vi "RVHR_Export Results_ExaPromPDF.vi"(6 "Local Data":T1, 7 "appended path":path, 8 "error in (no error)":errorcluster, 11 "Feature Table":string[][](array[string])=[["T1_KGN-MMK_LeftRail_20221114__0000000000.jpeg", "L", "Corrugation", "0.011096", "0.002368", "0.011096", "0.002368"], ["T1_KGN-MMK_LeftRail_20221114__0000000000.jpeg", "L", "Unknown", "0.012672", "0.001415", "0.013120", "0.001978"], ["T1_KGN-MMK_LeftRail_20221114__0000000000.jpeg", "L", "Unknown", "0.009825", "0.001763", "0.010158", "0.002166"], ["T1_KGN-MMK_RightRail_20221114__0000000000.jpeg", "R", "Unknown", "0.011674", "0.001198", "0.011674", "0.001198"], ["T1_KGN-MMK_RightRail_20221114__0000000000.jpeg", "R", "Unknown", "0.009925", "0.000982", "0.010548", "0.001386"], ["T1_KGN-MMK_LeftRail_20221114__0000000000.jpeg", "L", "Unknown", "0.001140", "0.000809", "-0.000002", "-0.000002"], ["T1_KGN-MMK_LeftRail_20221114__0000000000.jpeg", "L", "Unknown", "0.015532", "0.000852", "0.015532", "0.000852"], ["T1_KGN-MMK_RightRail_20221114__0000000000.jpeg", "R", "Unknown", "0.012845", "0.000938", "0.013062", "0.001184"], ["T1_KGN-MMK_RightRail_20221114__0000000000.jpeg", "R", "Corrugation", "0.009232", "0.000896", "0.009723", "0.001315"], ["T1_KGN-MMK_RightRail_20221114__0001500000.jpeg", "R", "Corrugation", "0.305360", "0.001430", "0.305880", "0.001834"], ["T1_KGN-MMK_LeftRail_20221114__0000000000.jpeg", "L", "Corrugation", "0.010821", "0.001661", "0.011428", "0.002166"], ["T1_KGN-MMK_LeftRail_20221114__0000000000.jpeg", "L", "Unknown", "0.010158", "0.000634", "0.010619", "0.000982"], ["T1_KGN-MMK_RightRail_20221114__0002000000.jpeg", "R", "Unknown", "0.408032", "0.001069", "0.408495", "0.001632"], ["T1_KGN-MMK_LeftRail_20221114__0002500000.jpeg", "L", "Unknown", "0.515705", "0.001372", "0.516241", "0.001863"], ["T1_KGN-MMK_RightRail_20221114__0002200000.jpeg", "R", "Unknown", "0.453206", "0.001140", "0.452628", "0.000867"]]) -> (0 "error out":errorcluster)   [LabVIEW 2024]
uses:
  Controls/RVHR - Local Data.ctl
  Controls/Test Cluster.ctl
  Controls/Excluded Information.ctl
  Controls/Language.ctl
  Controls/Device_Type.ctl
  <vilib>/Utility/miscctls.llb/LVRectTypeDef.ctl
  <vilib>/Utility/miscctls.llb/LVBoundsTypeDef.ctl
  <vilib>/Exaprom PDF/Controls/Initialization Controls/Captions.ctl
  <vilib>/Exaprom PDF/Controls/Initialization Controls/Image or Table Caption.ctl
  <vilib>/Exaprom PDF/Controls/Font Controls/Font complete cluster.ctl
  <vilib>/Exaprom PDF/Controls/Font Controls/Font size.ctl
  <vilib>/Exaprom PDF/Controls/Font Controls/Font color.ctl
  <vilib>/Exaprom PDF/Controls/Font Controls/Type and encoding.ctl
  <vilib>/Exaprom PDF/Controls/Text Controls/Unicode/Type and run direction.ctl
  <vilib>/Exaprom PDF/Controls/Initialization Controls/At the opening.ctl
  <vilib>/Exaprom PDF/Controls/Initialization Controls/Defaut Paragraphe and Line Spacing.ctl
  <vilib>/Exaprom PDF/Controls/Text Controls/Texte alignement.ctl
  <vilib>/Exaprom PDF/Controls/Text Controls/Line spacing.ctl
  <vilib>/Exaprom PDF/Controls/Page Controls/Page setup.ctl
  <vilib>/Exaprom PDF/Controls/Page Controls/Page size.ctl
  <vilib>/Exaprom PDF/Controls/Page Controls/Page Orientation.ctl
  <vilib>/Exaprom PDF/Controls/Page Controls/Page Layout Custom.ctl
  <vilib>/Exaprom PDF/Controls/Page Controls/Page margins.ctl
  <vilib>/Exaprom PDF/Controls/Initialization Controls/PDF Details.ctl
  <vilib>/Exaprom PDF/Controls/Initialization Controls/File Permission Parameters.ctl
  <vilib>/Exaprom PDF/Controls/Header, Footer and Watermark Controls/Header or Footer.ctl
  <vilib>/Exaprom PDF/Controls/Header, Footer and Watermark Controls/Header or Footer Line cluster.ctl
  <vilib>/Exaprom PDF/Controls/Header, Footer and Watermark Controls/Header Footer Line.ctl
  <vilib>/Exaprom PDF/Controls/Initialization Controls/Unit.ctl
  <vilib>/Exaprom PDF/Controls/Header, Footer and Watermark Controls/Header or Footer  Image cluster.ctl
  <vilib>/Exaprom PDF/Controls/Table Controls/Cell Alignment 20px.ctl
  <vilib>/Exaprom PDF/Controls/Table Controls/Table properties.ctl
  <vilib>/Exaprom PDF/Controls/Table Controls/Table position.ctl
  <vilib>/Exaprom PDF/Controls/Header, Footer and Watermark Controls/Header or Footer  Text cluster.ctl
  <vilib>/Exaprom PDF/Controls/Font Controls/Font complete cluster horizontal.ctl
  <vilib>/Exaprom PDF/Controls/Header, Footer and Watermark Controls/Header or Footer  Page # cluster.ctl
  <vilib>/Exaprom PDF/Controls/Header, Footer and Watermark Controls/Page number.ctl
  <vilib>/Exaprom PDF/Controls/Table Controls/Table Appearance and Font Row [ ].ctl
  <vilib>/Exaprom PDF/Controls/Table Controls/One Row Appearance.ctl
  <vilib>/Exaprom PDF/Controls/Table Controls/Row from to.ctl
  <vilib>/Exaprom PDF/Controls/Table Controls/Cell, Alignment, LS and Font - hide Vmerge.ctl
  <vilib>/Exaprom PDF/Controls/Table Controls/Cell Type, Alignment and LS.ctl
  <vilib>/Exaprom PDF/Controls/Table Controls/Text vertical arrangement.ctl
  <vilib>/Exaprom PDF/Controls/Table Controls/Cell Appearance.ctl
  <vilib>/Exaprom PDF/Controls/Table Controls/Cell Border 20 px.ctl
  <vilib>/Exaprom PDF/Controls/Table Controls/Merge Horizontal.ctl
  <vilib>/Exaprom PDF/Controls/Table Controls/Merge Vertical.ctl
  <vilib>/Exaprom PDF/VIs/Low level/Header, Footer and Watermark Low level/Append Text HF.vi
  <vilib>/Exaprom PDF/VIs/Low level/Header, Footer and Watermark Low level/AppendLine seperator.vi
  <vilib>/Exaprom PDF/VIs/Low level/Header, Footer and Watermark Low level/Append Image HF.vi
  <vilib>/Exaprom PDF/VIs/Low level/Header, Footer and Watermark Low level/Append Page number HF.vi
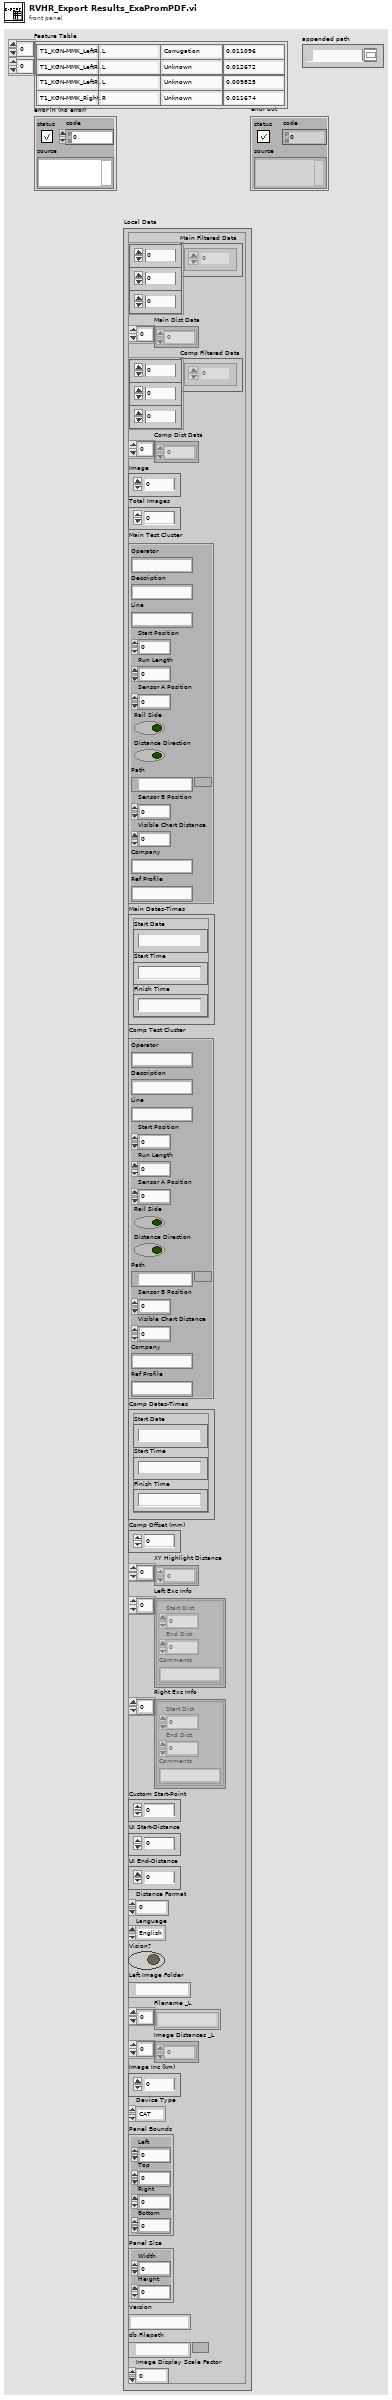
[diagram p1: front panel]
types:
  T1 = typedef "RVHR - Local Data.ctl" = cluster{"Main Filtered Data":dbl[][][], "Main Dist Data":dbl[], "Comp Filtered Data":dbl[][][], "Comp Dist Data":dbl[], "Image":u16, "Total Images":u16, "Main Test Cluster":T2, "Main Dates-Times":cluster{"Start Date":string, "Start Time":string, "Finish Time":string}, "Comp Test Cluster":T2, "Comp Dates-Times":cluster{"Start Date":string, "Start Time":string, "Finish Time":string}, "Comp Offset (mm)":i64, "XY Highlight Distance":dbl[], "Left Exc Info":T3[], "Right Exc Info":T3[], "Custom Start-Point":dbl, "UI Start-Distance":dbl, "UI End-Distance":dbl, "Distance Format":u8, "Language":T4, "Vision?":bool, "Left Image Folder":path, "Filename _L":string[], "Image Distances _L":dbl[], "Image Inc (km)":dbl, "Device Type":T5, "Panel Bounds":T6, "Panel Size":T7, "Version":string, "db Filepath":path, "Image Display Scale Factor":dbl}
  T2 = typedef "Test Cluster.ctl" = cluster{"Operator":string, "Description":string, "Line":string, "Start Position":dbl, "Run Length":dbl, "Sensor A Position":dbl, "Rail Side":bool, "Distance Direction":bool, "Path":path, "Sensor B Position":dbl, "Visible Chart Distance":dbl, "Company":string, "Ref Profile":string}
  T3 = typedef "Excluded Information.ctl" = cluster{"Start Dist":dbl, "End Dist":dbl, "Comments":string}
  T4 = typedef "Language.ctl" = enum16{"English", "Chinese", "German"}
  T5 = typedef "Device_Type.ctl" = enum16{"CAT", "Bi-CAT", "YRCA", "RCA", "RV-HR", "TV-HR"}
  T6 = typedef "LVRectTypeDef.ctl" = cluster{"Left":i16, "Top":i16, "Right":i16, "Bottom":i16}
  T7 = typedef "LVBoundsTypeDef.ctl" = cluster{"Width":u32, "Height":u32}
  T8 = typedef "Table Appearance and Font Row [ ].ctl" = T9[]
  T9 = typedef "One Row Appearance.ctl" = cluster{"Row":T10, "Cell [ ]":T11[]}
  T10 = typedef "Row from to.ctl" = cluster{"From #":i16, "to #":i16}
  T11 = typedef "Cell, Alignment, LS and Font - hide Vmerge.ctl" = cluster{"Text":T12, "Cell Appearance":T16, "HMerge":T18, "VMerge":T19, "Font":T20}
  T12 = typedef "Cell Type, Alignment and LS.ctl" = cluster{"Cell Alignment":T13, "Text rotation":T14, "Line spacing":T15}
  T13 = typedef "Cell Alignment 20px.ctl" = u16
  T14 = typedef "Text vertical arrangement.ctl" = enum16{"None", "Clockwise", "Counterclockwise"}
  T15 = typedef "Line spacing.ctl" = enum16{"Select", "1.0", "1.5", "2.0"}
  T16 = typedef "Cell Appearance.ctl" = cluster{"Border":T17, "Thickness":sgl, "Color":u32, "BG":u32}
  T17 = typedef "Cell Border 20 px.ctl" = u16
  T18 = typedef "Merge Horizontal.ctl" = cluster{"From":i8, "to":i8}
  T19 = typedef "Merge Vertical.ctl" = cluster{"From":i8, "to":i8}
  T20 = typedef "Font complete cluster.ctl" = cluster{"Name":string, "Size":T21, "Color":T22, "Style":cluster{"Bold":bool, "Italic":bool, "Underline":bool, "Strikeout":bool}, "Type":T23}
  T21 = typedef "Font size.ctl" = sgl
  T22 = typedef "Font color.ctl" = u32
  T23 = typedef "Type and encoding.ctl" = cluster{"Type&direction":T24, "Embedded":bool, "Encoding":string}
  T24 = typedef "Type and run direction.ctl" = enum16{"Select", "ASCII", "UTF-16", "UTF-16 (default)", "UTF-16 (LTR)", "UTF-16 (RTL)"}
  T25 = typedef "Table properties.ctl" = cluster{"Table position":T26, "SpacingBefore (points)":sgl, "SpacingAfter (points)":sgl}
  T26 = typedef "Table position.ctl" = i32
  T27 = typedef "Header or Footer  Text cluster.ctl" = cluster{"Start at page":i32, "Cell Alignment":T13, "Line spacing":T15, "Text":string, "Font complete":T28, "Link":string}
  T28 = typedef "Font complete cluster horizontal.ctl" = cluster{"Name":string, "Size":T21, "Color":T22, "Style":cluster{"Bold":bool, "Italic":bool, "Underline":bool, "Strikeout":bool}, "Type":T23}
  T29 = typedef "Header or Footer  Page # cluster.ctl" = cluster{"Start at page":i32, "Start with #":i32, "Cell Alignment":T13, "Page #":T30, "Font":T28}
  T30 = typedef "Page number.ctl" = cluster{"Text 1":string, "Text 2":string, "Text 3":string}
  T31 = typedef "Header or Footer.ctl" = enum16{"Header", "Footer"}
  T32 = typedef "Header or Footer  Image cluster.ctl" = cluster{"Start at page":i32, "Cell Alignment":T13, "Path":path, "Image (%)":sgl, "Link":string}
  T33 = typedef "Unit.ctl" = enum16{"inch", "mm"}
  T34 = typedef "Header or Footer Line cluster.ctl" = cluster{"H/F Line":T35, "Thickness (point)":sgl, " Colour":u32}
  T35 = typedef "Header Footer Line.ctl" = enum16{"No line", "Horizontal line"}
  T36 = typedef "File Permission Parameters.ctl" = cluster{"User Password":string, "Owner Password":string, "Printing":enum16{"Allow Printing", "Allow Degraded Printing", "Don't Allow Printing"}, "Allow Modify Contents":bool, "Allow Copy":bool, "Allow Modify Annotations":bool, "Allow Fill In ":bool, "Allow Screen Readers":bool, "Allow Assembly":bool}
  T37 = typedef "PDF Details.ctl" = cluster{"Title":string, "Author":string, "Subject":string, "Keywords":string, "Creator":string}
  T38 = typedef "Page setup.ctl" = cluster{"Page Size":T39, "Orientation":T40, "Custom Size":T41, "Margins":T42}
  T39 = typedef "Page size.ctl" = i32
  T40 = typedef "Page Orientation.ctl" = enum16{"Portrait", "Landscape"}
  T41 = typedef "Page Layout Custom.ctl" = cluster{"Width":sgl, "Height":sgl}
  T42 = typedef "Page margins.ctl" = cluster{"Left":sgl, "Right":sgl, "Top":sgl, "Bottom":sgl}
  T43 = typedef "Defaut Paragraphe and Line Spacing.ctl" = cluster{" Aligment":T44, "Line spacing":T15}
  T44 = typedef "Texte alignement.ctl" = enum16{"Select", "CENTER", "JUSTIFY", "LEFT", "RIGHT"}
  T45 = typedef "At the opening.ctl" = cluster{"Page":u16, "Show Bookmarks":bool}
  T46 = typedef "Captions.ctl" = cluster{"Figure":T47, "Table":T47, "Font":T20}
  T47 = typedef "Image or Table Caption.ctl" = cluster{"Caption":string, "Separator":string, "Position":enum16{"Above", "Below"}}
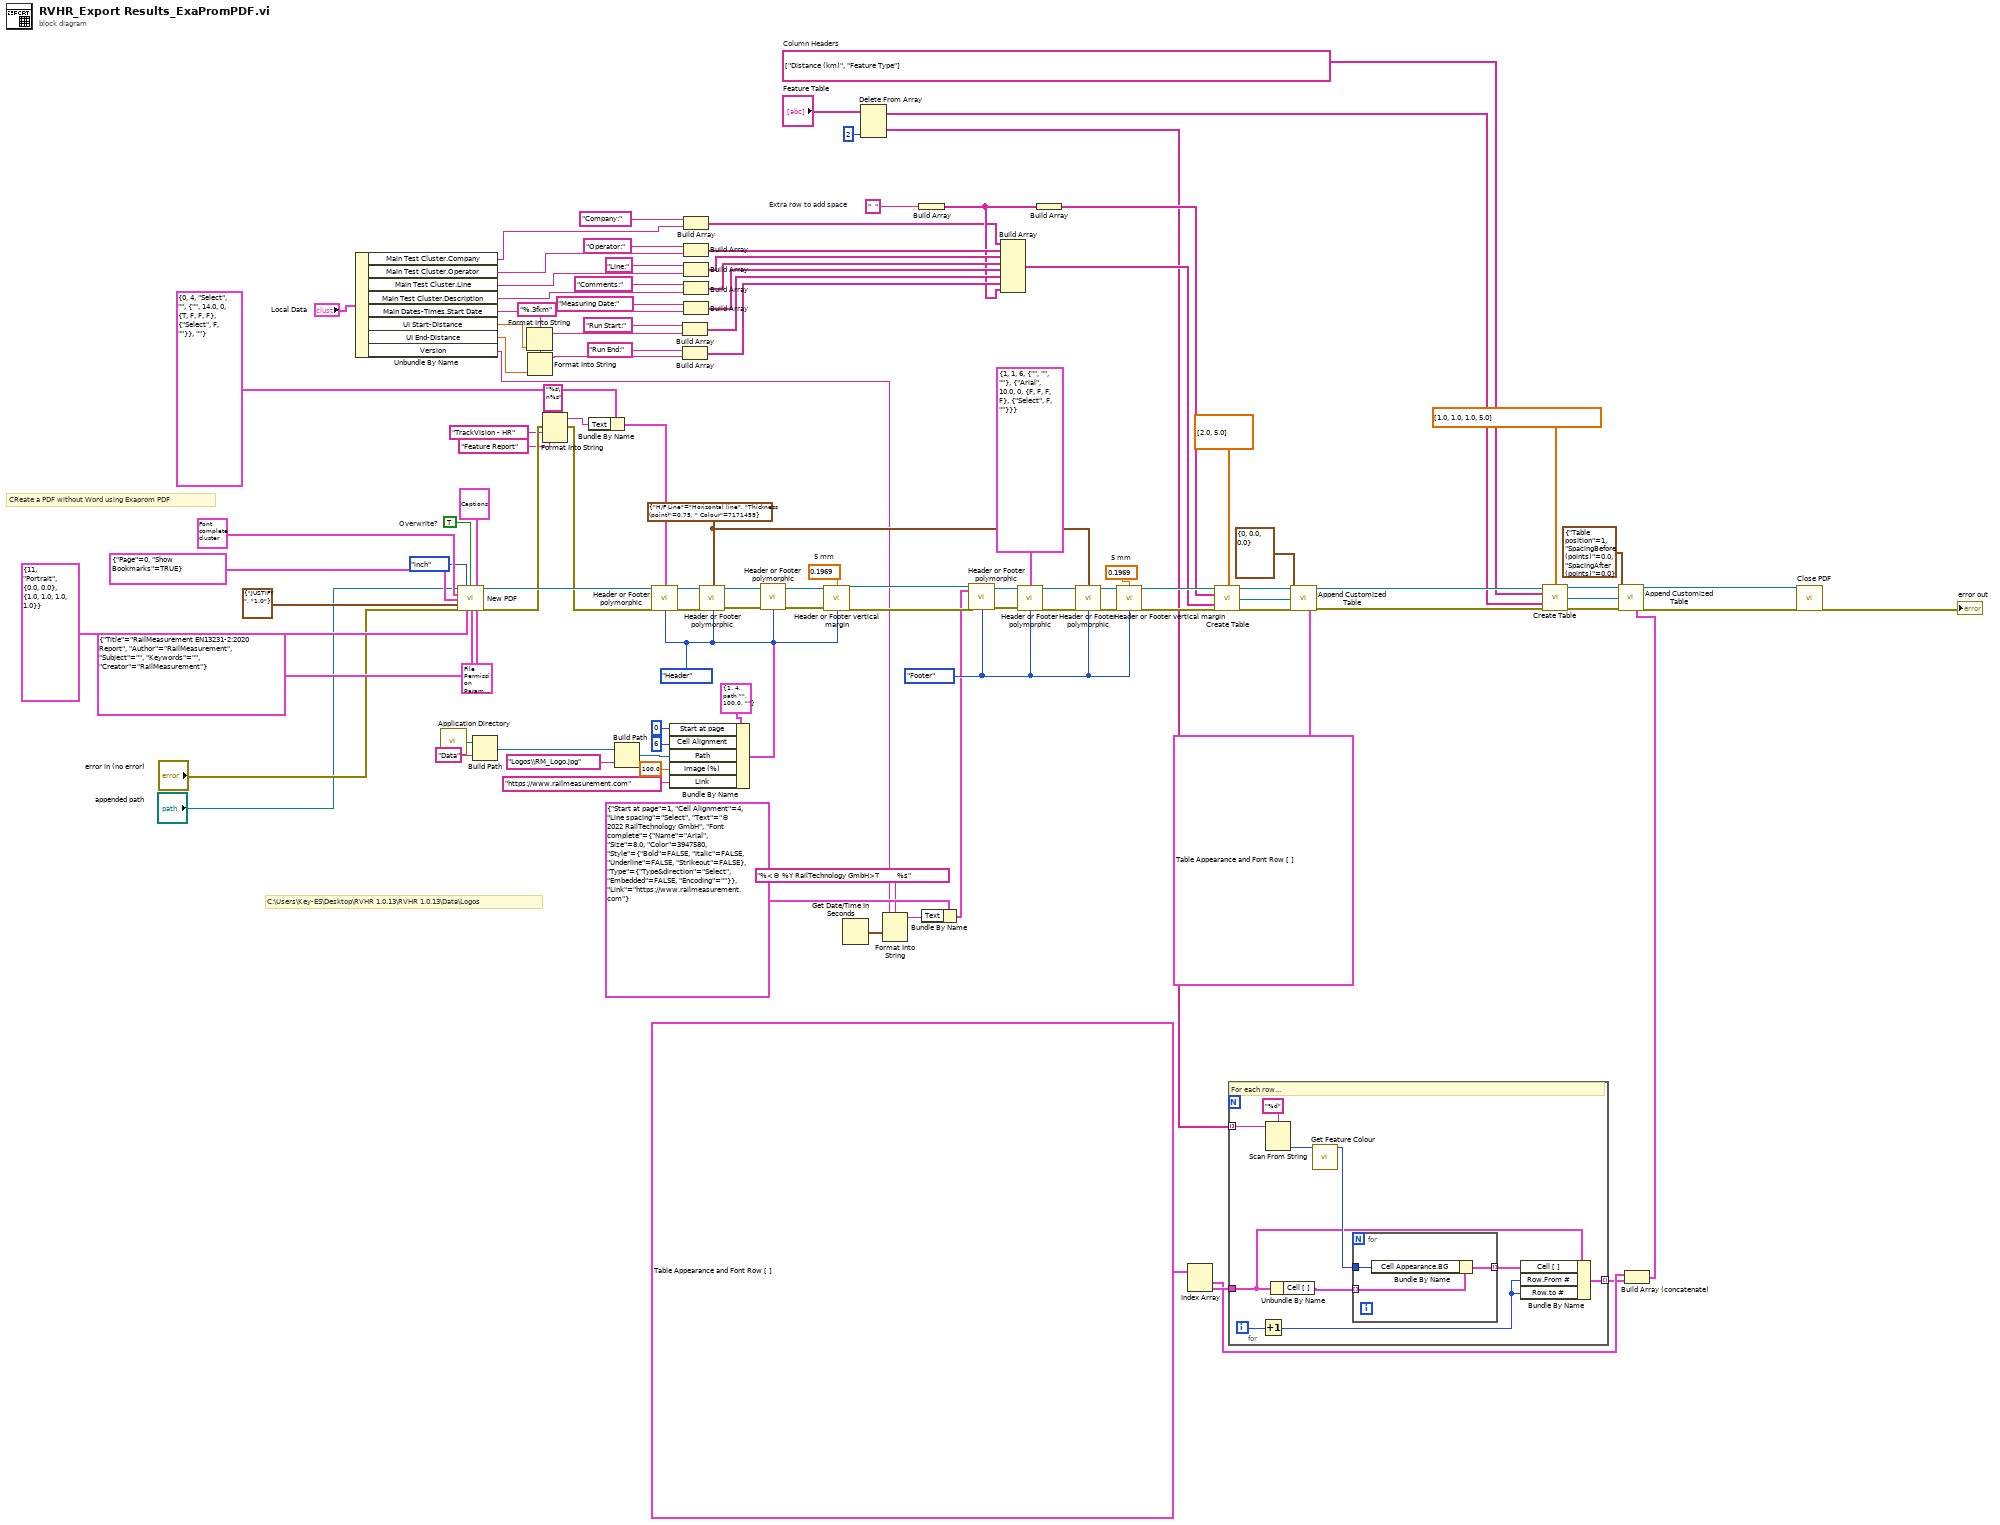
[diagram p0: block diagram]
diagram:
  w15 = "%.3fkm" ("format string")
  w26 = string[][] [["Distance (km)", "Feature Type"]]  # Column Headers
  w66 = "  "  # Extra row to add space
  w81 = 0.1969  # 5 mm
  w58 = Header_or_Footer."Footer" ("Position")
  w73 = T34 {"H/F Line"=enum."Horizontal line", "Thickness (point)"=0.75, " Colour"=7171459} ("Header Line")
  w105 = 0.1969  # 5 mm
  w96 = Header_or_Footer."Header" ("Position")
  w114 = TRUE  # Overwrite?
  # "C:\\Users\\Key-ES\\Desktop\\RVHR 1.0.13\\RVHR 1.0.13\\Data\\Logos"
  # "CReate a PDF without Word using Exaprom PDF"
  n1 = Unbundle By Name("Local Data") -> ("Main Test Cluster.Company"=w2:string, "Main Test Cluster.Operator"=w23:string, "Main Test Cluster.Line"=w22:string, "Main Test Cluster.Description"=w21:string, "Main Dates-Times.Start Date"=w20:string, "UI Start-Distance"=w19:dbl, "UI End-Distance"=w18:dbl, "Version"=w14:string)
  n2 = call <vilib>:"Application Directory.vi"() -> ("Application Directory"=w4:path)
  n3 = call <vilib>:"New PDF.vi"("PDF Path"="appended path", "Unit (default = mm)"=Unit."inch", "Overwrite?"=w114, "Captions"=T46 {"Figure"={"Caption"="Figure", "Separator"="  ", "Position"=enum."Below"}, "Table"={"Caption"="Table", "Separator"="  ", "Position"=enum."Above"}, "Font"={"Name"="", "Size"=-1.0, "Color"=0, "Style"={"Bold"=FALSE, "Italic"=FALSE, "Underline"=FALSE, "Strikeout"=FALSE}, "Type"={"Type&direction"=enum."Select", "Embedded"=FALSE, "Encoding"=""}}}, "Default Font"=T20 {"Name"="Arial", "Size"=12.0, "Color"=0, "Style"={"Bold"=FALSE, "Italic"=FALSE, "Underline"=FALSE, "Strikeout"=FALSE}, "Type"={"Type&direction"=enum."ASCII", "Embedded"=FALSE, "Encoding"=""}}, "At the opening"=T45 {"Page"=0, "Show Bookmarks"=TRUE}, "Default Paragraph"=T43 {" Aligment"=enum."JUSTIFY", "Line spacing"=enum."1.0"}, "error in (no error)"="error in (no error)", "Page Setup"=T38 {"Page Size"=11, "Orientation"=enum."Portrait", "Custom Size"={"Width"=0.0, "Height"=0.0}, "Margins"={"Left"=1.0, "Right"=1.0, "Top"=1.0, "Bottom"=1.0}}, "PDF Details"=T37 {"Title"="RailMeasurement EN13231-2:2020 Report", "Author"="RailMeasurement", "Subject"="", "Keywords"="", "Creator"="RailMeasurement"}, "Permissions"=T36 {"User Password"="", "Owner Password"="", "Printing"=enum."Allow Printing", "Allow Modify Contents"=TRUE, "Allow Copy"=TRUE, "Allow Modify Annotations"=TRUE, "Allow Fill In "=TRUE, "Allow Screen Readers"=TRUE, "Allow Assembly"=TRUE}) -> ("PDF Report"=w102:refnum<class "PDF Report Class.lvclass">, "error out"=w68:errorcluster)  [unwired: 3 out]
  n4 = Build Path(base path=w4, name or relative path="Data") -> (appended path=w90:path)
  n5 = Format Into String(format string=w15, w19) -> (resulting string=w16:string)  [unwired: 2 in, 1 out]
  n6 = Format Into String(format string=w15, w18) -> (resulting string=w17:string)  [unwired: 2 in, 1 out]
  n7 = Format Into String(format string="%s\n%s", error in=w68, "TrackVision - HR" ("input 1"), "Feature Report" ("input 2")) -> (resulting string=w71:string, error out=w67:errorcluster)  [unwired: 1 in]
  n8 = Bundle By Name(cluster=T27 {"Start at page"=0, "Cell Alignment"=4, "Line spacing"=enum."Select", "Text"="", "Font complete"={"Name"="", "Size"=14.0, "Color"=0, "Style"={"Bold"=TRUE, "Italic"=FALSE, "Underline"=FALSE, "Strikeout"=FALSE}, "Type"={"Type&direction"=enum."Select", "Embedded"=FALSE, "Encoding"=""}}, "Link"=""} ("Header Text"), "Text"=w71) -> (w69:T27)
  n9 = Build Path(base path=w90, name or relative path="Logos\\RM_Logo.jpg") -> (appended path=w53:path)
  n10 = call-poly <vilib>:"Header or Footer polymorphic.vi"("PDF Report IN"=w102, "Header or footer"=w69, "error in (no error)"=w67, "Position"=w96) -> ("PDF Report OUT"=w104:refnum<class "PDF Report Class.lvclass">, "error out"=w103:errorcluster)  [unwired: 10 out]
  n11 = Bundle By Name(cluster=T32 {"Start at page"=1, "Cell Alignment"=4, "Path"=path "", "Image (%)"=100.0, "Link"=""} ("Header or footer"), "Start at page"=0, "Cell Alignment"=T13 6, "Path"=w53, "Image (%)"=sgl 100.0, "Link"="https://www.railmeasurement.com") -> (w94:T32)
  n12 = Build Array("Run Start:" ("element"), w16) -> (w42:string[])
  n13 = Build Array("Run End:" ("element"), w17) -> (w41:string[])
  n14 = Build Array("Company:" ("element"), w2) -> (w1:string[])
  n15 = Build Array("Operator:" ("element"), w23) -> (w48:string[])
  n16 = Build Array("Line:" ("element"), w22) -> (w46:string[])
  n17 = Build Array("Comments:" ("element"), w21) -> (w47:string[])
  n18 = Build Array("Measuring Date:" ("element"), w20) -> (w43:string[])
  n19 = call-poly <vilib>:"Header or Footer polymorphic.vi"("PDF Report IN"=w104, "H/F Line"=w73, "error in (no error)"=w103, "Position"=w96) -> ("PDF Report OUT"=w100:refnum<class "PDF Report Class.lvclass">, "error out"=w99:errorcluster)  [unwired: 1 in, 9 out]
  n20 = call-poly <vilib>:"Header or Footer polymorphic.vi"("PDF Report IN"=w100, "Header or footer"=w94, "error in (no error)"=w99, "Position"=w96) -> ("PDF Report OUT"=w97:refnum<class "PDF Report Class.lvclass">, "error out"=w98:errorcluster)  [unwired: 1 in, 9 out]
  n21 = call <vilib>:"Header or Footer vertical margin.vi"("PDF Report IN"=w97, "Vertical margin"=w105, "error in (no error)"=w98, "Position"=w96) -> ("PDF Report OUT"=w62:refnum<class "PDF Report Class.lvclass">, "error out"=w61:errorcluster)  [unwired: 10 out]
  n22 = Get Date/Time In Seconds() -> (seconds since 1Jan1904=w54:timestamp)
  n23 = Delete From Array(array="Feature Table", index (col)=2 ("disabled index (col)")) -> (deleted portion=w5:string[], array with subset deleted=w6:string[][])  [unwired: 2 in]
  n24 = Format Into String(format string="%<© %Y RailTechnology GmbH>T         %s", w54, w14) -> (resulting string=w55:string)  [unwired: 2 in, 1 out]
  n25 = Build Array(w66) -> (w25:string[])
  n26 = Bundle By Name(cluster=T27 {"Start at page"=1, "Cell Alignment"=4, "Line spacing"=enum."Select", "Text"="© 2022 RailTechnology GmbH", "Font complete"={"Name"="Arial", "Size"=8.0, "Color"=3947580, "Style"={"Bold"=FALSE, "Italic"=FALSE, "Underline"=FALSE, "Strikeout"=FALSE}, "Type"={"Type&direction"=enum."Select", "Embedded"=FALSE, "Encoding"=""}}, "Link"="https://www.railmeasurement.com"} ("Footer Text"), "Text"=w55) -> (w57:T27)
  n27 = call-poly <vilib>:"Header or Footer polymorphic.vi"("PDF Report IN"=w62, "Header or footer"=w57, "error in (no error)"=w61, "Position"=w58) -> ("PDF Report OUT"=w59:refnum<class "PDF Report Class.lvclass">, "error out"=w60:errorcluster)  [unwired: 10 out]
  n28 = Build Array(w1, w48, w46, w47, w43, w42, w41, w25) -> (w40:string[][])
  n29 = call-poly <vilib>:"Header or Footer polymorphic.vi"("PDF Report IN"=w59, "Header or footer"=T29 {"Start at page"=1, "Start with #"=1, "Cell Alignment"=6, "Page #"={"Text 1"="", "Text 2"="", "Text 3"=""}, "Font"={"Name"="Arial", "Size"=10.0, "Color"=0, "Style"={"Bold"=FALSE, "Italic"=FALSE, "Underline"=FALSE, "Strikeout"=FALSE}, "Type"={"Type&direction"=enum."Select", "Embedded"=FALSE, "Encoding"=""}}} ("Footer Page #"), "error in (no error)"=w60, "Position"=w58) -> ("PDF Report OUT"=w77:refnum<class "PDF Report Class.lvclass">, "error out"=w76:errorcluster)  [unwired: 10 out]
  n30 = Build Array(w25) -> (w65:string[][])
  n31 = call-poly <vilib>:"Header or Footer polymorphic.vi"("PDF Report IN"=w77, "H/F Line"=w73, "error in (no error)"=w76, "Position"=w58) -> ("PDF Report OUT"=w74:refnum<class "PDF Report Class.lvclass">, "error out"=w75:errorcluster)  [unwired: 1 in, 9 out]
  n32 = call <vilib>:"Header or Footer vertical margin.vi"("PDF Report IN"=w74, "Vertical margin"=w81, "error in (no error)"=w75, "Position"=w58) -> ("PDF Report OUT"=w78:refnum<class "PDF Report Class.lvclass">, "error out"=w79:errorcluster)  [unwired: 10 out]
  n33 = Index Array(array=T8 [{"Row"={"From #"=0, "to #"=0}, "Cell [ ]"=[{"Text"={"Cell Alignment"=5, "Text rotation"=enum."None", "Line spacing"=enum."Select"}, "Cell Appearance"={"Border"=5, "Thickness"=0.5, "Color"=0, "BG"=16777225}, "HMerge"={"From"=-1, "to"=-1}, "VMerge"={"From"=-1, "to"=-1}, "Font"={"Name"="", "Size"=10.0, "Color"=0, "Style"={"Bold"=TRUE, "Italic"=FALSE, "Underline"=FALSE, "Strikeout"=FALSE}, "Type"={"Type&direction"=enum."Select", "Embedded"=FALSE, "Encoding"=""}}}, {"Text"={"Cell Alignment"=5, "Text rotation"=enum."None", "Line spacing"=enum."Select"}, "Cell Appearance"={"Border"=5, "Thickness"=0.5, "Color"=0, "BG"=16777225}, "HMerge"={"From"=-1, "to"=-1}, "VMerge"={"From"=-1, "to"=-1}, "Font"={"Name"="", "Size"=10.0, "Color"=0, "Style"={"Bold"=TRUE, "Italic"=FALSE, "Underline"=FALSE, "Strikeout"=FALSE}, "Type"={"Type&direction"=enum."Select", "Embedded"=FALSE, "Encoding"=""}}}]}, {"Row"={"From #"=1, "to #"=-1}, "Cell [ ]"=[{"Text"={"Cell Alignment"=5, "Text rotation"=enum."None", "Line spacing"=enum."Select"}, "Cell Appearance"={"Border"=5, "Thickness"=0.5, "Color"=0, "BG"=16777225}, "HMerge"={"From"=-1, "to"=-1}, "VMerge"={"From"=-1, "to"=-1}, "Font"={"Name"="", "Size"=10.0, "Color"=0, "Style"={"Bold"=FALSE, "Italic"=FALSE, "Underline"=FALSE, "Strikeout"=FALSE}, "Type"={"Type&direction"=enum."Select", "Embedded"=FALSE, "Encoding"=""}}}, {"Text"={"Cell Alignment"=5, "Text rotation"=enum."None", "Line spacing"=enum."Select"}, "Cell Appearance"={"Border"=5, "Thickness"=0.5, "Color"=0, "BG"=16777225}, "HMerge"={"From"=-1, "to"=-1}, "VMerge"={"From"=-1, "to"=-1}, "Font"={"Name"="", "Size"=10.0, "Color"=0, "Style"={"Bold"=FALSE, "Italic"=FALSE, "Underline"=FALSE, "Strikeout"=FALSE}, "Type"={"Type&direction"=enum."Select", "Embedded"=FALSE, "Encoding"=""}}}]}] ("Row  [ ]")) -> (element #1=w11:T9, element #2=w12:T9)  [unwired: 2 in]
  n34 = call <vilib>:"Create Table.vi"("PDF Report IN"=w78, "Table columnWidth [ ]"=sgl[] [2.0, 5.0], "Column Headers 2D [ ]"=w65, "Text Data 2D [ ]"=w40, "error in (no error)"=w79) -> ("PDF Report duplicate"=w84:refnum<class "PDF Report Class.lvclass">, "PDF Table"=w85:refnum<class "Pdfp Table Class.lvclass">, "error out"=w86:errorcluster)  [unwired: 8 in]
  n35 = for {
    tunnel: w12 -> [w116]
    tunnel: [w115] -> w10 mode=indexing
    tunnel: w5 -> [w123] mode=indexing
    i -> [w118]
    # "For each row..."
    n36 = Increment(x=w118) -> (x+1=w117:i32)
    n37 = Scan From String(format string="%d", input string=w123) -> (output 1=w122:u16)  [unwired: 3 in, 3 out]
    n38 = Unbundle By Name(w116) -> ("Cell [ ]"=w121:T11[])
    n39 = call "Get Feature Colour.vi"("Feature Type"=w122) -> ("color"=w120:u32)  [unwired: 10 in]
    n40 = for {
      tunnel: w121 -> [w127] mode=indexing
      tunnel: w120 -> [w126]
      tunnel: [w125] -> w119 mode=indexing
      n41 = Bundle By Name(cluster=w127, "Cell Appearance.BG"=w126) -> (w125:T11)
    }
    n42 = Bundle By Name(cluster=w116, "Cell [ ]"=w119, "Row.From #"=w117, "Row.to #"=w117) -> (w115:T9)
  }
  n43 = call <vilib>:"Append Customized Table.vi"("PDF Report IN"=w84, "Table properties"=T25 {"Table position"=0, "SpacingBefore (points)"=0.0, "SpacingAfter (points)"=0.0}, "PDF Table"=w85, "error in (no error)"=w86, "Row  [ ]"=T8 [{"Row"={"From #"=0, "to #"=-2}, "Cell [ ]"=[{"Text"={"Cell Alignment"=4, "Text rotation"=enum."None", "Line spacing"=enum."Select"}, "Cell Appearance"={"Border"=0, "Thickness"=0.5, "Color"=0, "BG"=16777225}, "HMerge"={"From"=-1, "to"=-1}, "VMerge"={"From"=-1, "to"=-1}, "Font"={"Name"="", "Size"=-1.0, "Color"=0, "Style"={"Bold"=FALSE, "Italic"=FALSE, "Underline"=FALSE, "Strikeout"=FALSE}, "Type"={"Type&direction"=enum."Select", "Embedded"=FALSE, "Encoding"=""}}}, {"Text"={"Cell Alignment"=4, "Text rotation"=enum."None", "Line spacing"=enum."Select"}, "Cell Appearance"={"Border"=0, "Thickness"=0.5, "Color"=0, "BG"=16777225}, "HMerge"={"From"=-1, "to"=-1}, "VMerge"={"From"=-1, "to"=-1}, "Font"={"Name"="", "Size"=-1.0, "Color"=0, "Style"={"Bold"=FALSE, "Italic"=FALSE, "Underline"=FALSE, "Strikeout"=FALSE}, "Type"={"Type&direction"=enum."Select", "Embedded"=FALSE, "Encoding"=""}}}]}]) -> ("PDF Report OUT"=w27:refnum<class "PDF Report Class.lvclass">, "error out"=w28:errorcluster)  [unwired: 9 in]
  n44 = call <vilib>:"Create Table.vi"("PDF Report IN"=w27, "Table columnWidth [ ]"=sgl[] [1.0, 1.0, 1.0, 5.0], "Column Headers 2D [ ]"=w26, "Text Data 2D [ ]"=w6, "error in (no error)"=w28) -> ("PDF Report duplicate"=w33:refnum<class "PDF Report Class.lvclass">, "PDF Table"=w32:refnum<class "Pdfp Table Class.lvclass">, "error out"=w31:errorcluster)  [unwired: 8 in]
  n45 = Build Array (concatenate)(w11, w10) -> (w9:T9[])
  n46 = call <vilib>:"Append Customized Table.vi"("PDF Report IN"=w33, "Table properties"=T25 {"Table position"=1, "SpacingBefore (points)"=0.0, "SpacingAfter (points)"=0.0}, "PDF Table"=w32, "error in (no error)"=w31, "Row  [ ]"=w9) -> ("PDF Report OUT"=w30:refnum<class "PDF Report Class.lvclass">, "error out"=w29:errorcluster)  [unwired: 9 in]
  n47 = call <vilib>:"Close PDF.vi"("PDF Report"=w30, "error in (no error)"=w29) -> ("error out"=→"error out":errorcluster)  [unwired: 13 out]
